vi "createSerialCommunicator.vi"(8 "error in (no error)":errorcluster, 10 "Serial Protocol":T1, 11 "ISerialCommFactory in":refnum<class "ISerialCommFactory.lvclass">) -> (0 "error out":errorcluster, 2 "serialCommunicator":refnum<class "SerialCommunicator.lvclass">, 3 "ISerialCommFactory out":refnum<class "ISerialCommFactory.lvclass">)   [LabVIEW 2013, in "SerialProtocols.lvlib" / "ISerialCommFactory.lvclass"]
uses:
  <userlib>/Common/SerialProtocols/SerialCommFactory/ISerialCommFactory/ISerialCommFactory.lvclass
  <userlib>/Common/SerialProtocols/SerialCommunicator/SerialCommunicator/SerialCommunicator.lvclass
  <userlib>/Common/SerialProtocols/Configuration/SerialProtocol.ctl
  <userlib>/Common/SerialProtocols/SerialProtocols.lvlib
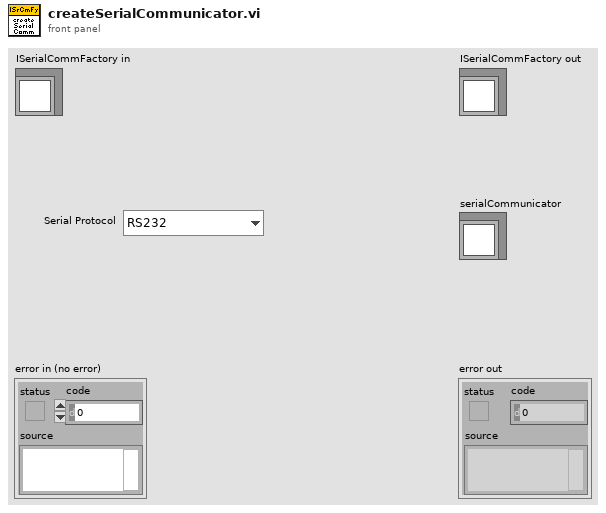
[diagram p1: front panel]
types:
  T1 = typedef "SerialProtocols.lvlib/SerialProtocol.ctl" = enum16{"RS232", "RS485", "SerialSimulator"}
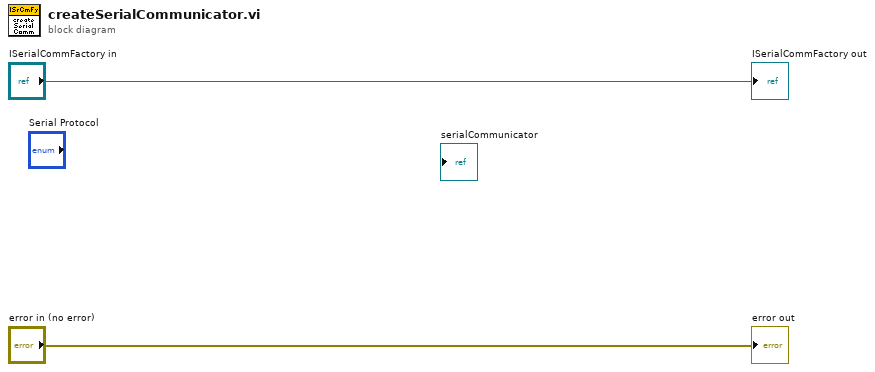
[diagram p0: block diagram]
diagram:
  "error out" <- "error in (no error)"
  "ISerialCommFactory out" <- "ISerialCommFactory in"
